vi "main.vi"   [LabVIEW 2025]
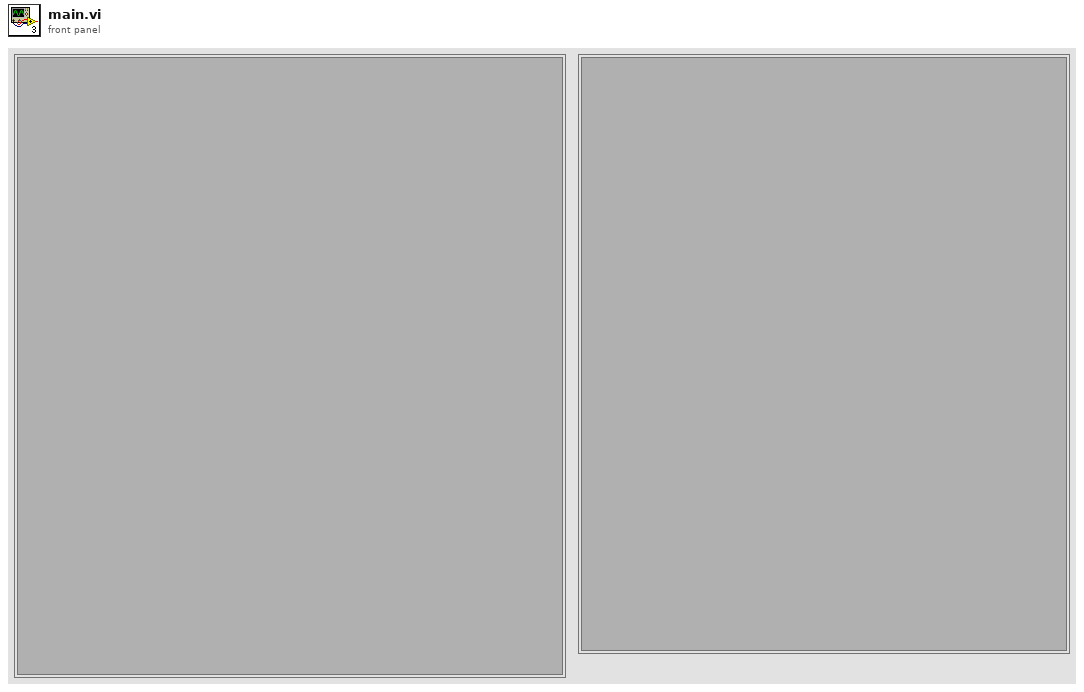
[diagram p1: front panel]
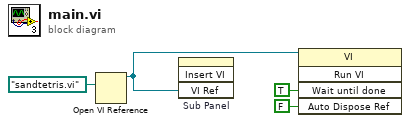
[diagram p0: block diagram]
diagram:
  n1 = Open VI Reference(vi path=path "sandtetris.vi") -> (vi reference=w4:refnum<vi>)  [unwired: 5 in, 1 out]
  n2 = invoke on="Sub Panel" class="SubPnl" method="Insert VI"("VI Ref"=w4) -> ()  [unwired: 3 in, 4 out]
  n3 = invoke class="VI" method="Run VI"(reference=w4, "Wait until done"=TRUE ("Wait Until Done"), "Auto Dispose Ref"=FALSE ("Auto Dispose Reference")) -> ()  [unwired: 2 in, 5 out]
